vi "DFD FXP Code Generator_OBS_v75.vi"   [LabVIEW 2017, in "NI_DigFilterLicensed.lvlib"]
doc: "Generates only fixed-point integer code for a fixed-point filter, without generating floating-point code. You can use this polymorphic VI to generate LabVIEW code or C code. You can select the polymorphic instance manually."
uses:
  <vilib>/addons/Digital Filter Design/NI_DigFilterLicensed.lvlib
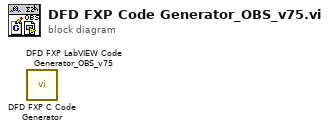
[diagram p0: block diagram]
diagram:
  n1 = call <vilib>:"DFD FXP C Code Generator.vi"() -> ()  [unwired: 10 in, 2 out]
  n2 = call <vilib>:"DFD FXP LabVIEW Code Generator_OBS_v75.vi"() -> ()  [unwired: 10 in, 2 out]
